vi "Actor Core.vi"(8 "error in":errorcluster, 11 "Nested in":refnum<class "F Generator.lvclass">) -> (0 "error out":errorcluster, 3 "Actor out":refnum<class "Actor.lvclass">)   [LabVIEW 2020, in "F Generator.lvlib" / "F Generator.lvclass"]
doc: "(<B>Filename</B>: Actor Framework.lvlib:Actor.lvclass:Actor Core.vi)\n\nReceives messages to the actor, reacts to them, and initiates any error handling that may shut the actor down.\n\nDescendant classes may override this VI to append parallel tasks for the actor to complete while it handles messages. Overrides use the Call Parent Method node."
uses:
  F Generator.lvclass
  C:/Program Files/National Instruments/LabVIEW 2020/vi.lib/ActorFramework/Actor/Actor.lvclass
  <vilib>/ActorFramework/Actor/Actor.lvclass
  Measurement GEN/Measurement GEN.lvclass
  F Generator.lvclass/F Generator.ctl
  <vilib>/ActorFramework/Actor/Actor.lvclass/Actor.ctl
  <vilib>/ActorFramework/Message Enqueuer/Message Enqueuer.lvclass/Message Enqueuer.ctl
  F Generator Messages/Start Stop graph Msg/Start Stop graph Msg.lvclass/Start Stop graph Msg.ctl
  F Generator Messages/Log Enable Msg/Log Enable Msg.lvclass/Log Enable Msg.ctl
  F Generator Messages/File path Msg/File path Msg.lvclass/File path Msg.ctl
  F Generator Messages/Select Format File Msg/Select Format File Msg.lvclass/Select Format File Msg.ctl
  F Generator Messages/Amplitud Msg/Amplitud Msg.lvclass/Amplitud Msg.ctl
  F Generator Messages/Frecuencia Msg/Frecuencia Msg.lvclass/Frecuencia Msg.ctl
  <vilib>/ActorFramework/Message Enqueuer/Init from Existing Queue.vi
  <vilib>/ActorFramework/Message Enqueuer/Enqueue.vi
  <vilib>/ActorFramework/Stop Msg/Stop Msg.lvclass
  C:/Program Files/National Instruments/LabVIEW 2020/vi.lib/ActorFramework/Message/Message.lvclass
  F Generator Messages/Start Stop graph Msg/Start Stop graph Msg.lvclass
  F Generator Messages/Log Enable Msg/Log Enable Msg.lvclass
  F Generator Messages/File path Msg/File path Msg.lvclass
  F Generator Messages/Select Format File Msg/Select Format File Msg.lvclass
  F Generator Messages/Amplitud Msg/Amplitud Msg.lvclass
  F Generator Messages/Frecuencia Msg/Frecuencia Msg.lvclass
  <vilib>/ActorFramework/Message Priority Queue/Priority Enqueue.vi
  <vilib>/ActorFramework/Message Enqueuer/Message Enqueuer.lvclass
panel:
  out "Waveform Chart":waveform(dbl)(graph)
  in  "Tipo Señal":T1(ring)
  in  "Frecuencia":dbl(slide) scale=0.0..100.0
  in  "Amplitud":dbl(slide) scale=0.0..10.0
  in  "Formato":enum16{"tdms", "txt", "csv"}(ring)
  in  "File Path":path
  in  "Save":bool
  in  "Stop":bool
  in  "Start":bool
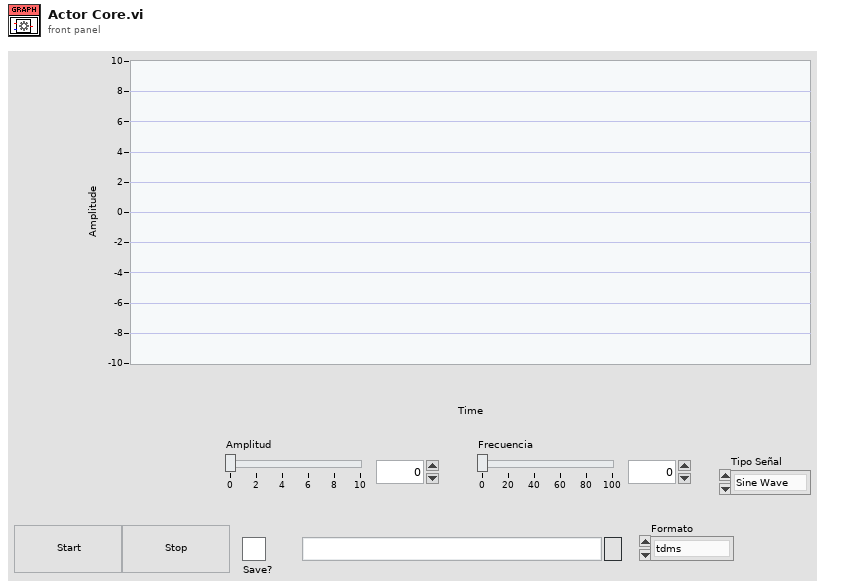
[diagram p1: front panel]
types:
  T1 = enum16{"Sine Wave", "Triangle Wave", "Square Wave", "Sawtooth Wave"}
  T2 = enum8{"Enabled", "Disabled", "Disabled and Grayed Out"}
  T3 = cluster{"Stop":refnum<user-event>, "WF Chart":refnum<user-event>}
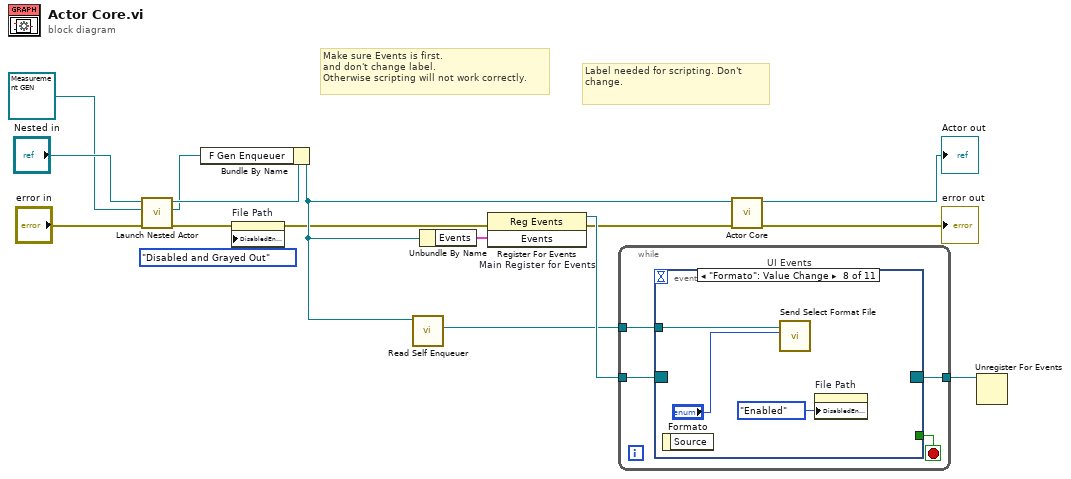
[diagram p0: block diagram]
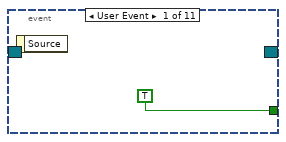
[diagram p2: hidden frame]
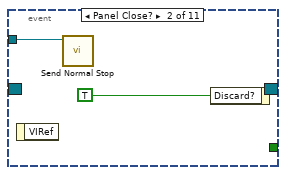
[diagram p3: hidden frame]
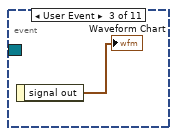
[diagram p4: hidden frame]
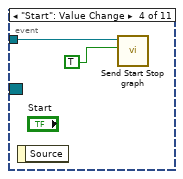
[diagram p5: hidden frame]
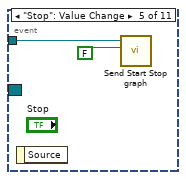
[diagram p6: hidden frame]
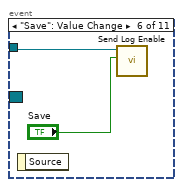
[diagram p7: hidden frame]
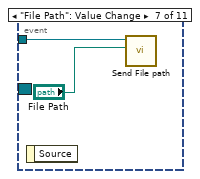
[diagram p8: hidden frame]
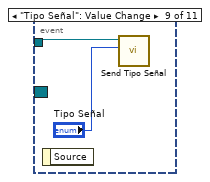
[diagram p9: hidden frame]
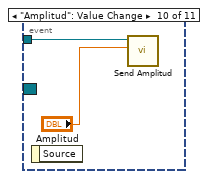
[diagram p10: hidden frame]
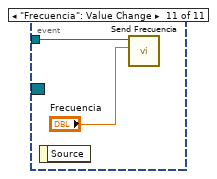
[diagram p11: hidden frame]
diagram:
  # "Label needed for scripting. Don't change."
  # "Make sure Events is first.\nand don't change label.\nOtherwise scripting will not work correctly."
  n1 = call <vilib>:"Launch Nested Actor.vi"("error in (no error)"="error in", "Nested Actor"=refnum<class "Measurement GEN.lvclass"> refnum ("Measurement GEN.lvlib:Measurement GEN.lvclass"), "Caller Actor in"="Nested in") -> ("error out"=w1:errorcluster, "Nested Actor's Enqueuer"=w4:refnum<class "Message Enqueuer.lvclass">, "Caller Actor out"=w7:refnum<class "F Generator.lvclass">)  [unwired: 6 in]
  n2 = Bundle By Name(cluster=w7, "F Gen Enqueuer"=w4) -> (w5:refnum<class "F Generator.lvclass">)
  n3 = property on="File Path" class="Path"(error in=w1, "DisabledEnum"=T2."Disabled and Grayed Out" ("Disabled")) -> (error out=w2:errorcluster)  [unwired: 1 in, 1 out]
  n4 = call <vilib>:"Read Self Enqueuer.vi"("Actor"=w5) -> ("Self Enqueuer"=w11:refnum<class "Message Enqueuer.lvclass">)  [unwired: 10 in]
  n5 = Unbundle By Name(w5) -> ("Events"=w13:T3)
  n6 = register-events "Main Register for Events"(error in=w2, w13) -> (reference out=w14:refnum<event-registration>, error out=w9:errorcluster)  [unwired: 1 in]
  n7 = while {
    tunnel: w14 -> [w20]
    tunnel: [w18] -> w12
    tunnel: w11 -> [w17]
    stop <- w19 stop-if-true
    n8 = event "UI Events" shown="[7] \"Formato\": Value Change" {
      selector: w20 -> [_ _ _ _ _ _ _ _ _ _ _]
      dyn-events: [_ _ _ _ _ _ _ _ _ _ _] -> w18
      timeout: _ -> [_ _ _ _ _ _ _ _ _ _ _]
      tunnel: [TRUE _ _ _ _ _ _ _ _ _ _] -> w19
      tunnel: w17 -> [_ w22 _ w26 w28 w29 w32 w35 w37 w39 w41]
      event User Event {
        n9 = event-data() -> ()  [unwired: 1 in, 1 out]
      }
      event Panel Close? {
        n10 = event-data() -> ()  [unwired: 1 in, 1 out]
        n11 = call <vilib>:"Send Normal Stop.vi"("Message Enqueuer"=w22) -> ()  [unwired: 10 in, 1 out]
        n12 = event-data("Discard?"=TRUE) -> ()  [unwired: 1 in, 1 out]
      }
      event User Event {
        n13 = event-data() -> ("signal out"=→"Waveform Chart":waveform(dbl))  [unwired: 1 in]
      }
      event "Start": Value Change {
        n14 = event-data() -> ()  [unwired: 1 in, 1 out]
        n15 = call "Send Start Stop graph.vi"("Start/Stop"=TRUE, "Message Enqueuer"=w26) -> ()  [unwired: 8 in, 2 out]
      }
      event "Stop": Value Change {
        n16 = event-data() -> ()  [unwired: 1 in, 1 out]
        n17 = call "Send Start Stop graph.vi"("Start/Stop"=FALSE, "Message Enqueuer"=w28) -> ()  [unwired: 8 in, 2 out]
      }
      event "Save": Value Change {
        n18 = event-data() -> ()  [unwired: 1 in, 1 out]
        n19 = call "Send Log Enable.vi"("Log Enable?"="Save", "Message Enqueuer"=w29) -> ()  [unwired: 8 in, 2 out]
      }
      event "File Path": Value Change {
        n20 = event-data() -> ()  [unwired: 1 in, 1 out]
        n21 = call "Send File path.vi"("File Path"="File Path", "Message Enqueuer"=w32) -> ()  [unwired: 8 in, 2 out]
      }
      event "Formato": Value Change {
        n22 = event-data() -> ()  [unwired: 1 in, 1 out]
        n23 = call "Send Select Format File.vi"("Formato"="Formato", "Message Enqueuer"=w35) -> ()  [unwired: 8 in, 2 out]
        n24 = property on="File Path" class="Path"("DisabledEnum"=T2."Enabled" ("Disabled")) -> ()  [unwired: 2 in, 2 out]
      }
      event "Tipo Señal": Value Change {
        n25 = event-data() -> ()  [unwired: 1 in, 1 out]
        n26 = call "Send Tipo Señal.vi"("Tipo Señal"="Tipo Señal", "Message Enqueuer"=w37) -> ()  [unwired: 8 in, 2 out]
      }
      event "Amplitud": Value Change {
        n27 = event-data() -> ()  [unwired: 1 in, 1 out]
        n28 = call "Send Amplitud.vi"("Amplitud"="Amplitud", "Message Enqueuer"=w39) -> ()  [unwired: 8 in, 2 out]
      }
      event "Frecuencia": Value Change {
        n29 = event-data() -> ()  [unwired: 1 in, 1 out]
        n30 = call "Send Frecuencia.vi"("Frecuencia"="Frecuencia", "Message Enqueuer"=w41) -> ()  [unwired: 8 in, 2 out]
      }
    }
  }
  n31 = call-parent "Actor Core.vi"("error in"=w9, "Actor in"=w5) -> ("error out"=→"error out":errorcluster, "Actor out"=→"Actor out":refnum<class "Actor.lvclass">)  [unwired: 8 in]
  n32 = Unregister For Events(event registration refnum=w12) -> ()  [unwired: 1 in, 1 out]
